vi "Sub VI simulador captura dado.vi"(6 "error constant":errorcluster) -> (4 "error constant 2":errorcluster, 5 "Dato capturado":dbl)   [LabVIEW 2020]
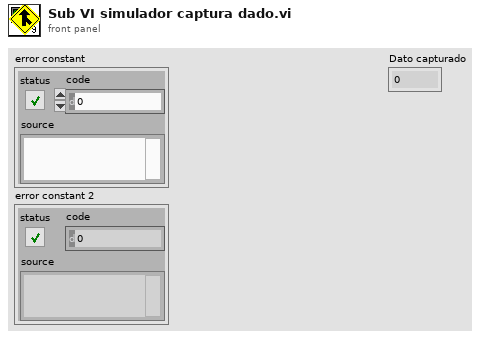
[diagram p1: front panel]
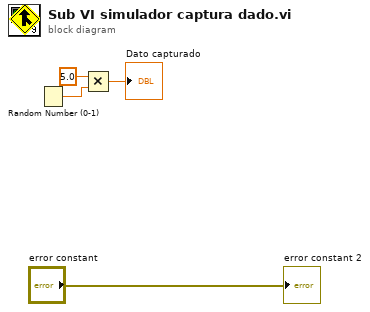
[diagram p0: block diagram]
diagram:
  n1 = Random Number (0-1)() -> (number: 0 to 1=w3:dbl)
  n2 = Multiply(x=5.0, y=w3) -> (x*y=→"Dato capturado":dbl)
  "error constant 2" <- "error constant"
